vi "movement forward by santimeters.vi"(5 "I2C Ref in":T1, 8 "error in (no error)":errorcluster, 11 "distance (cm)":dbl format="%#_13g") -> (0 "error out":errorcluster, 2 "I2C Ref out":T1)   [LabVIEW 2017]
uses:
  <vilib>/myRIO/Instrument Drivers/Onboard IO/I2C/typedefs/I2C Reference.ctl
  <vilib>/myRIO/Common/Instrument Driver Framework/Utilities/typedefs/myRIO Generic Hardware Reference.ctl
  <vilib>/myRIO/Common/Instrument Driver Framework/Utilities/typedefs/Hardware Version Enum.ctl
  <vilib>/myRIO/Common/Instrument Driver Framework/Utilities/typedefs/myRIO v1.0 Reference.ctl
  <vilib>/myRIO/Common/Instrument Driver Framework/Utilities/typedefs/Generic FPGA Reference.ctl
  <vilib>/myRIO/Common/Instrument Driver Framework/myRIO v1.0/I2C/typedefs/I2C Channels Enum.ctl
  <vilib>/myRIO/Instrument Drivers/Onboard IO/I2C/typedefs/I2C Configuration.ctl
  <vilib>/myRIO/Instrument Drivers/Onboard IO/I2C/typedefs/I2C Transfer Rate.ctl
  <vilib>/myRIO/Common/Instrument Driver Framework/myRIO v1.0/Encoder/typedefs/Encoder Signal Mode.ctl
  <vilib>/myRIO/Instrument Drivers/Onboard IO/Encoder/typedefs/Encoder Reference.ctl
  <vilib>/myRIO/Common/Instrument Driver Framework/myRIO v1.0/Encoder/typedefs/Encoder Channels Enum.ctl
  <vilib>/myRIO/Common/Instrument Driver Framework/myRIO v1.0/Encoder/typedefs/Encoder Configuration v1.0.ctl
  <vilib>/userdefined/High Color/nirio_resource_hc.ctl
  <vilib>/myRIO/Common/Instrument Driver Framework/Utilities/vis/Is FPGA Ref Available.vi
  <vilib>/myRIO/Common/Instrument Driver Framework/myRIO v1.0/Encoder/vis/myRIO v1.1 Open Encoder.vi
  <vilib>/myRIO/Instrument Drivers/Onboard IO/Encoder/vis/Read.vi
  <vilib>/myRIO/Common/Instrument Driver Framework/Utilities/vis/Validate Channels.vi
  <vilib>/myRIO/Common/Instrument Driver Framework/myRIO v1.0/Encoder/vis/myRIO v1.0 Reserve Encoder.vi
  <vilib>/myRIO/Common/Instrument Driver Framework/myRIO v1.0/Encoder/vis/myRIO v1.0 Build MUX Configuration Encoder.vi
  <vilib>/myRIO/Common/Instrument Driver Framework/myRIO v1.0/Resource Manager/vis/myRIO v1.0 Reserve Channel List.vi
  <vilib>/myRIO/Common/Instrument Driver Framework/myRIO v1.0/Resource Manager/vis/myRIO v1.0 Create Configuration List.vi
  <vilib>/myRIO/Common/Instrument Driver Framework/myRIO v1.0/Resource Manager/vis/myRIO v1.0 Reserve Channel.vi
  <vilib>/myRIO/Common/Instrument Driver Framework/myRIO v1.0/Resource Manager/vis/myRIO v1.0 Unreserve Channel.vi
  <vilib>/myRIO/Common/Instrument Driver Framework/myRIO v1.0/Resource Manager/vis/myRIO v1.0 Build Mutex Name.vi
  <vilib>/Utility/VariantDataType/GetNumericInfo.vi
  <vilib>/Utility/error.llb/Error Cluster From Error Code.vi
  <vilib>/myRIO/Common/Instrument Driver Framework/myRIO v1.0/myRIO v1.1 Open.vi
  <vilib>/myRIO/Common/Instrument Driver Framework/Utilities/vis/IO Manager.vi
  <vilib>/myRIO/Common/Instrument Driver Framework/Utilities/vis/Configuration Manager.vi
  <vilib>/myRIO/Common/Instrument Driver Framework/myRIO v1.0/Resource Manager/vis/myRIO v1.0 Configure IO.vi
  <vilib>/myRIO/Common/Instrument Driver Framework/myRIO v1.0/myRIO v1.0 Close.vi
  <vilib>/myRIO/Common/Instrument Driver Framework/myRIO v1.0/Encoder/vis/myRIO v1.0 Configure Encoder.vi
  <vilib>/myRIO/Common/Instrument Driver Framework/myRIO v1.0/Encoder/vis/myRIO v1.0 Read Encoder.vi
  <vilib>/myRIO/Common/Instrument Driver Framework/myRIO v1.0/DIO/vis/myRIO v1.0 Write DIO.vi
  <vilib>/myRIO/Express VI/Onboard IO/Encoder/Encoder Express VI.xnode
  <vilib>/myRIO/Instrument Drivers/Onboard IO/Encoder/vis/myRIO Encoder Open.xnode
  <vilib>/myRIO/Instrument Drivers/Onboard IO/Encoder/Encoder.lvlib
  <vilib>/myRIO/Instrument Drivers/Onboard IO/DIO/DIO.lvlib
  <vilib>/myRIO/Instrument Drivers/Onboard IO/I2C/I2C.lvlib
panel:
  out "main angle":ext
  out "axis Z(after)":ext
  out "zero angle":ext
  out "left":dbl
  out "right":dbl
  out "axis Z(paste)":ext
  in  "Stop Button":bool
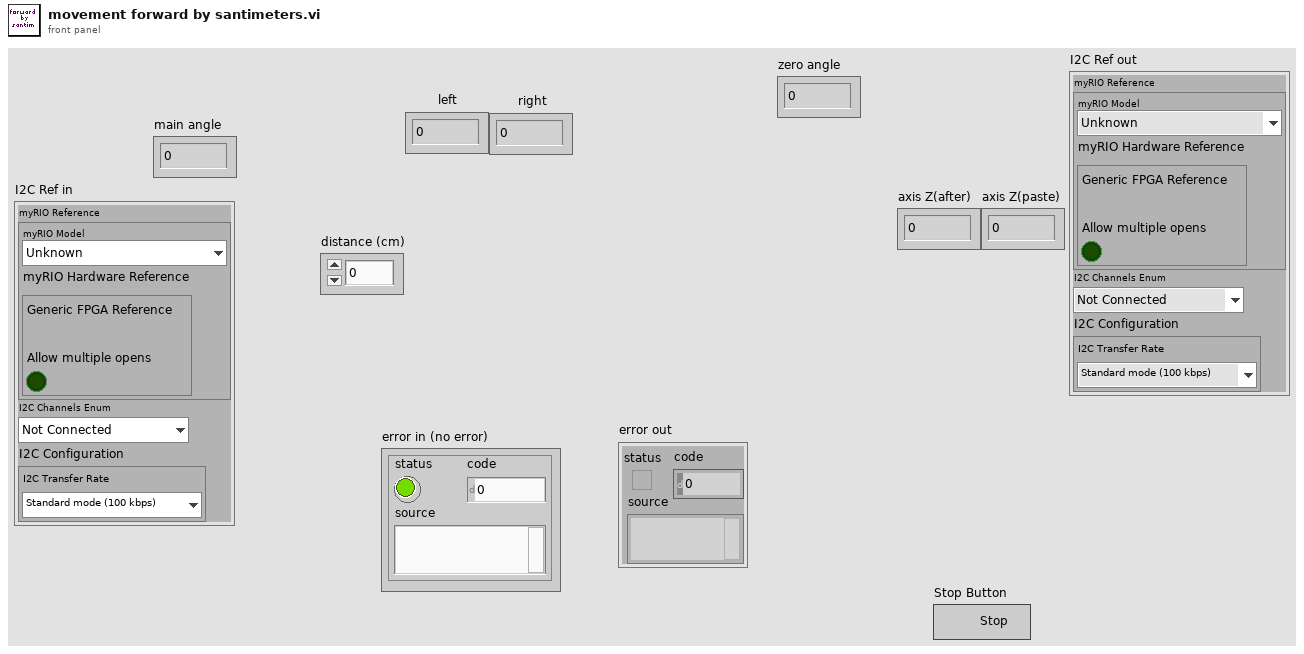
[diagram p1: front panel]
types:
  T1 = typedef "I2C.lvlib/I2C Reference.ctl" = cluster{"myRIO Reference":T2, "I2C Channels Enum":T6, "I2C Configuration":T7}
  T2 = typedef "myRIO Generic Hardware Reference.ctl" = cluster{"myRIO Model":T3, "myRIO Hardware Reference":T4}
  T3 = typedef "Hardware Version Enum.ctl" = enum16{"Unknown", "myRIO-1900", "myRIO-1950", "roboRIO", "NI ELVIS RIO CM"}
  T4 = typedef "myRIO v1.0 Reference.ctl" = cluster{"Generic FPGA Reference":T5, "Allow multiple opens":bool}
  T5 = typedef "Generic FPGA Reference.ctl" = refnum<k20>
  T6 = typedef "I2C Channels Enum.ctl" = enum16{"Not Connected", "A/I2C", "B/I2C", "I2C/I2C"}
  T7 = typedef "I2C.lvlib/I2C Configuration.ctl" = cluster{"I2C Transfer Rate":T8}
  T8 = typedef "I2C.lvlib/I2C Transfer Rate.ctl" = enum16{"Standard mode (100 kbps)", "Fast mode (400 kbps)"}
  T9 = typedef "DIO.lvlib/DIO Reference.ctl" = cluster{"myRIO Reference":T2, "DIO Channels List":T10}
  T10 = typedef "DIO Channels List.ctl" = T11[]
  T11 = typedef "DIO Channels Enum.ctl" = enum16{"Not Connected", "C/DIO0", "C/DIO1", "C/DIO2", "C/DIO3", "C/DIO4", "C/DIO5", "C/DIO6", "C/DIO7", "A/DIO0", "A/DIO1", "A/DIO2", "A/DIO3", "A/DIO4", "A/DIO5", "A/DIO6", "A/DIO7", "A/DIO8", "A/DIO9", "A/DIO10", "A/DIO11", "A/DIO12", "A/DIO13", "A/DIO14", "A/DIO15", "B/DIO0", "B/DIO1", "B/DIO2", "B/DIO3", "B/DIO4", "B/DIO5", "B/DIO6", "B/DIO7", "B/DIO8", "B/DIO9", "B/DIO10", "B/DIO11", "B/DIO12", "B/DIO13", "B/DIO14", "B/DIO15", "LED0", "LED1", "LED2", "LED3", "Button0", "DIO/DIO0", "DIO/DIO1", "DIO/DIO2", "DIO/DIO3", "DIO/DIO4", "DIO/DIO5", "DIO/DIO6", "DIO/DIO7", "DIO/DIO8", "DIO/DIO9", "SPI/CS0", "SPI/CS1", "SPI/CS2", "SPI/CS3", "LED RADIO (Green)", "LED RADIO (Red)", "LED COMM (Green)", "LED COMM (Red)", "LED MODE (Green)", "LED MODE (Red)"}
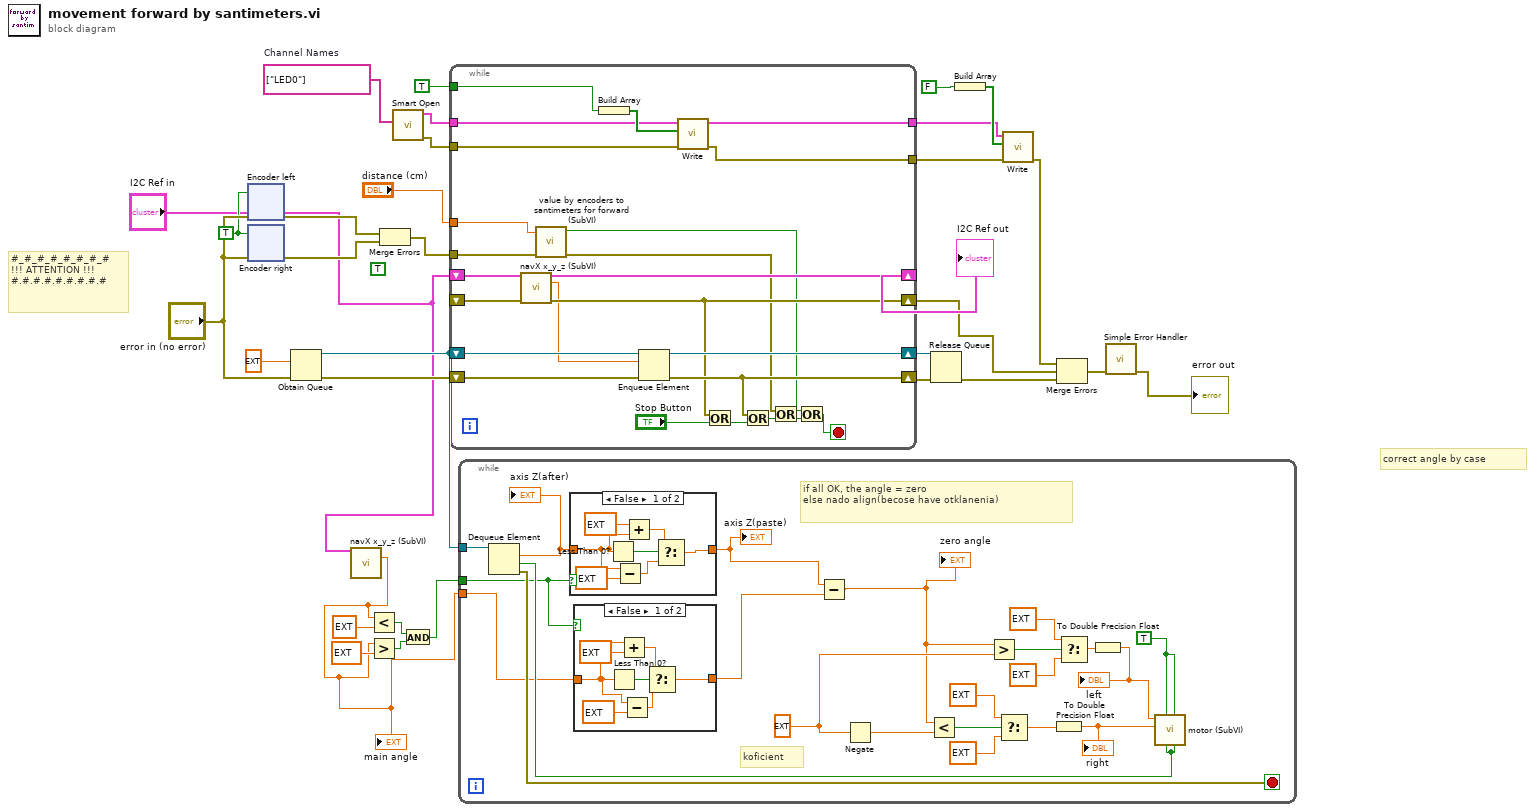
[diagram p0: block diagram]
diagram:
  w11 = tag[] ["LED0"]  # Channel Names
  w12 = TRUE ("Reset Counter")
  (unwired) TRUE ("Allow multiple opens?")
  # "correct angle by case"
  # "#_#_#_#_#_#_#_#\n!!! ATTENTION !!!\n#.#.#.#.#.#.#.#.#"
  n1 = xnode ("Encoder left")("error in (no error)"="error in (no error)", "Reset Counter"=w12) -> ("error out"=w16:errorcluster)  [unwired: 3 out]
  n2 = xnode ("Encoder right")("error in (no error)"="error in (no error)", "Reset Counter"=w12) -> ("error out"=w15:errorcluster)  [unwired: 3 out]
  n3 = Obtain Queue(element data type=ext 0.0 ("value Z"), error in (no error)="error in (no error)") -> (queue out=w25:refnum<queue>, error out=w32:errorcluster)  [unwired: 3 in, 1 out]
  n4 = call "navX x_y_z (SubVI).vi"("I2C Ref Out in"="I2C Ref in") -> ("value Z"=w21:ext)  [unwired: 10 in, 4 out]
  "main angle" <- w21
  n5 = Less?(x=w21, y=ext 90.0) -> (x < y?=w19:bool)
  n6 = Greater?(x=w21, y=ext -90.0) -> (0:w22:bool)
  n7 = Merge Errors(w16, w15) -> (w14:errorcluster)
  n8 = call <vilib>:"Smart Open.vi"("Channel Names"=w11) -> ("error out"=w6:errorcluster, "DIO Ref Out"=w7:T9)  [unwired: 9 in]
  n9 = And(x=w19, y=w22) -> (x .and. y?=w18:bool)
  n10 = while {
    shift-right: [w50] -> w30
    shift-left: w32 -> [w55]
    shift-right: [w54] -> w31
    shift-left: w25 -> [w56]
    shift-right: [w51] -> w28
    shift-left: "I2C Ref in" -> [w52]
    shift-right: [w47] -> w1
    shift-left: _ -> [w48]
    tunnel: w14 -> [w42]
    tunnel: "distance (cm)" -> [w40]
    tunnel: TRUE -> [w37]
    tunnel: w7 -> [w36]
    tunnel: w6 -> [w35]
    tunnel: [w34] -> w4
    tunnel: [w33] -> w5
    stop <- w44 stop-if-true
    n11 = call "navX x_y_z (SubVI).vi"("I2C Ref Out in"=w52, "error in (no error)"=w48) -> ("I2C Ref Out out"=w51:T1, "value Z"=w46:ext, "error out"=w47:errorcluster)  [unwired: 9 in, 2 out]
    n12 = call "value by encoders to santimeters for forward (SubVI).vi"("error in (no error)"=w42, "range in"=w40) -> ("error out"=w41:errorcluster, "value >= range"=w39:bool)  [unwired: 7 in, 1 out]
    n13 = Build Array(w37) -> (w38:bool[])
    n14 = Enqueue Element(queue=w56, element=w46, error in (no error)=w55) -> (queue out=w54:refnum<queue>, error out=w50:errorcluster)  [unwired: 1 in, 1 out]
    n15 = call <vilib>:"Write.vi"("error in (no error)"=w35, "Values"=w38, "DIO Ref In"=w36) -> ("error out"=w33:errorcluster, "DIO Ref Out"=w34:T9)  [unwired: 6 in]
    n16 = Or(x=w47, y="Stop Button") -> (x .or. y?=w49:bool)
    n17 = Or(x=w50, y=w49) -> (x .or. y?=w45:bool)
    n18 = Or(x=w41, y=w45) -> (x .or. y?=w43:bool)
    n19 = Or(x=w39, y=w43) -> (x .or. y?=w44:bool)
  }
  "I2C Ref out" <- w28
  n20 = while {
    tunnel: w25 -> [w78]
    tunnel: w21 -> [w60]
    tunnel: w18 -> [w59]
    stop <- w77 stop-if-true
    w66 = TRUE ("M0 (Pin 21)")
    w70 = ext 1.0 ("y")
    # "koficient"
    # "if all OK, the angle = zero\nelse nado align(becose have otklanenia)"
    n21 = Dequeue Element(queue=w78) -> (element=w62:ext, timed out?=w65:bool, error out=w77:errorcluster)  [unwired: 2 in, 1 out]
    "axis Z(after)" <- w62
    n22 = case shown="False" w59 {
      tunnel: [w92 w94] -> w63
      tunnel: w62 -> [w88 w94]
      frame False {
        n23 = Less Than 0?(x=w88) -> (x < 0?=w93:bool)
        n24 = Subtract(x=w88, y=ext 180.0) -> (x-y=w89:ext)
        n25 = Add(x=ext 180.0, y=w88) -> (x+y=w91:ext)
        n26 = Select(t=w91, s=w93, f=w89) -> (s? t:f=w92:ext)
      }
      frame True {
      }
    }
    "axis Z(paste)" <- w63
    n27 = case shown="False" w59 {
      tunnel: [w84 w86] -> w61
      tunnel: w60 -> [w81 w86]
      frame False {
        n28 = Less Than 0?(x=w81) -> (x < 0?=w85:bool)
        n29 = Add(x=w81, y=ext 180.0) -> (x+y=w83:ext)
        n30 = Subtract(x=w81, y=ext 180.0) -> (x-y=w82:ext)
        n31 = Select(t=w83, s=w85, f=w82) -> (s? t:f=w84:ext)
      }
      frame True {
      }
    }
    n32 = Subtract(x=w63, y=w61) -> (x-y=w64:ext)
    "zero angle" <- w64
    n33 = Negate(x=w70) -> (-x=w69:ext)
    n34 = Less?(x=w64, y=w69) -> (x < y?=w73:bool)
    n35 = Greater?(x=w64, y=w70) -> (0:w76:bool)
    n36 = Select(t=ext 0.2 ("y"), s=w73, f=ext 0.30000000000000000001 ("y")) -> (s? t:f=w67:ext)
    n37 = To Double Precision Float(number=w67) -> (double precision float=w58:dbl)
    "right" <- w58
    n38 = Select(t=ext 0.2 ("y"), s=w76, f=ext 0.30000000000000000001 ("y")) -> (s? t:f=w68:ext)
    n39 = To Double Precision Float(number=w68) -> (double precision float=w57:dbl)
    "left" <- w57
    n40 = call "motor (SubVI).vi"("M1 (Pin 26)"=w65, "M1 (Pin 25)"=w66, "M0 (Pin 23)"=w65, "M0 (Pin 21)"=w66, "PWM1"=w58, "PWM0"=w57) -> ()  [unwired: 5 in, 1 out]
  }
  n41 = Release Queue(queue=w31, error in (no error)=w30) -> (error out=w26:errorcluster)  [unwired: 1 in, 2 out]
  n42 = Build Array(FALSE) -> (w10:bool[])
  n43 = call <vilib>:"Write.vi"("error in (no error)"=w5, "Values"=w10, "DIO Ref In"=w4) -> ("error out"=w3:errorcluster)  [unwired: 6 in, 1 out]
  n44 = Merge Errors(w3, w1, w26) -> (w27:errorcluster)
  n45 = call <vilib>:"Simple Error Handler.vi"("error in (no error)"=w27) -> ("error out"=→"error out":errorcluster)  [unwired: 4 in, 4 out]
